vi "Tabla_multiplicar.vi"() -> ()   [LabVIEW 2020]
panel:
  out "Índice":dbl
  in  "Renglón":dbl
  in  "Columna":dbl
  in  "Columnas":dbl
  in  "Renglones":dbl
  out "Arreglo de multiplicación":dbl[][](array[numeric])
  # "Configuración del tamaño del arreglo"
  # "Índice del elemento"
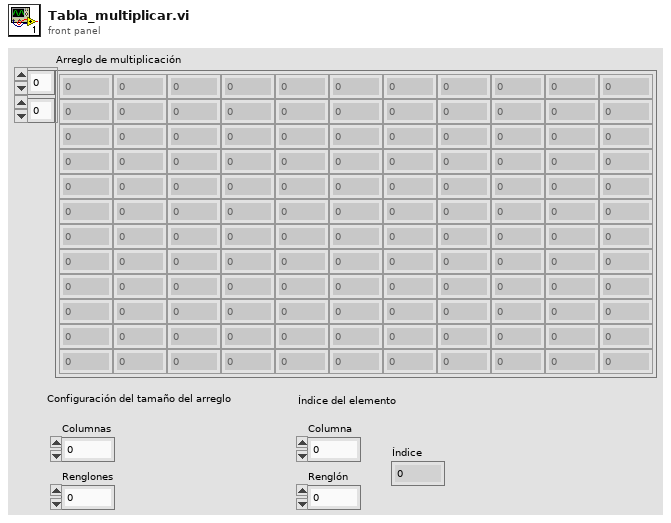
[diagram p1: front panel]
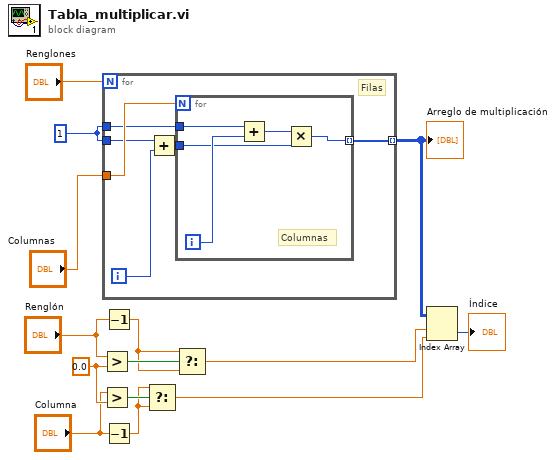
[diagram p0: block diagram]
diagram:
  w10 = 0.0
  w12 = 1
  n1 = Greater?(x="Renglón", y=w10) -> (0:w8:bool)
  n2 = Greater?(x="Columna", y=w10) -> (0:w9:bool)
  n3 = for {
    N: "Renglones" -> [_]
    tunnel: "Columnas" -> [w20]
    tunnel: w12 -> [w18]
    tunnel: w12 -> [w17]
    tunnel: [w15] -> w11 mode=indexing
    i -> [w19]
    # "Filas"
    n4 = Add(x=w17, y=w19) -> (x+y=w16:i32)
    n5 = for {
      N: w20 -> [_]
      tunnel: w18 -> [w24]
      tunnel: w16 -> [w22]
      tunnel: [w21] -> w15 mode=indexing
      i -> [w25]
      # "Columnas"
      n6 = Add(x=w24, y=w25) -> (x+y=w23:i32)
      n7 = Multiply(x=w23, y=w22) -> (x*y=w21:i32)
    }
  }
  "Arreglo de multiplicación" <- w11
  n8 = Decrement(x="Renglón") -> (x-1=w2:dbl)
  n9 = Decrement(x="Columna") -> (x-1=w1:dbl)
  n10 = Select(t=w1, s=w9, f=w1) -> (s? t:f=w5:dbl)
  n11 = Select(t=w2, s=w8, f=w2) -> (s? t:f=w4:dbl)
  n12 = Index Array(array=w11, index (row)=w4, index (col)=w5) -> (element=→"Índice":i32)
